vi "DataCollectWithTimeout.vi"(7 "Notifier Data":T2, 8 "error in (no error)":errorcluster, 9 "Timeout":dbl=5.0, 10 "Data Cluster":T1, 11 "Notifier in":refnum<notifier>) -> (0 "error out":errorcluster, 1 "Free Air Flow Data":dbl[][](array[numeric]), 2 "STOP Button Pressed":bool, 3 "Free Air Flow Measurement Complete":bool, 4 "Vacuum Data":dbl, 5 "Air Flow Data":dbl)   [LabVIEW 2026, in "Acquisition.lvlib"]
uses:
  Acquisition.lvlib
  controls/NotifierAndDataQueue.ctl
  controls/WaveformChartData.ctl
  Hardware Configuration.ctl
  Settings/Settings.lvlib
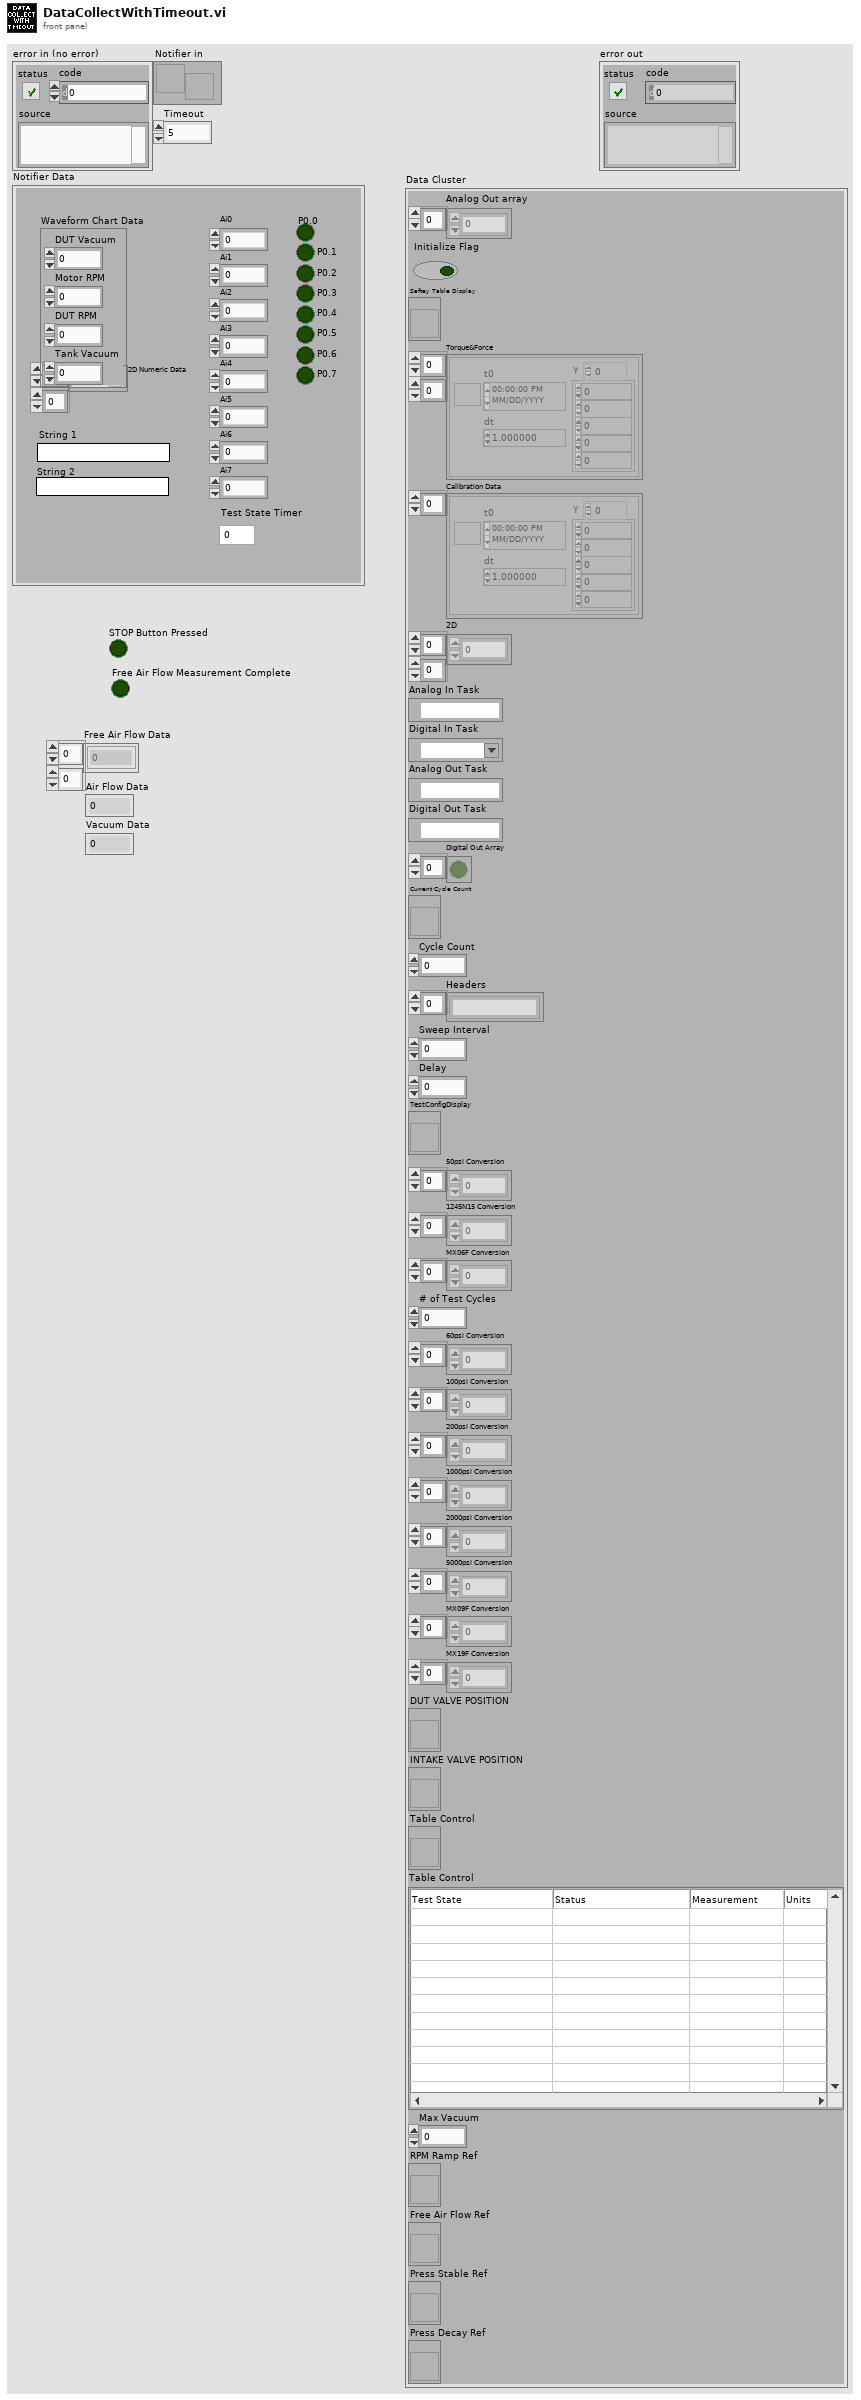
[diagram p1: front panel]
types:
  T1 = typedef "Acquisition.lvlib/Hardware Configuration.ctl" = cluster{"Analog Out array":dbl[], "Initialize Flag":bool, "Saftey Table Display":refnum<vi>, "Torque&Force":waveform(dbl)[][], "Calibration Data":waveform(dbl)[], "2D":dbl[][], "Analog In Task":refnum<k21>, "Digital In Task":refnum<k21>, "Analog Out Task":refnum<k21>, "Digital Out Task":refnum<k21>, "Digital Out Array":bool[], "Current Cycle Count":refnum<vi>, "Cycle Count":u64, "Headers":string[], "Sweep Interval":u64, "Delay":u64, "TestConfigDisplay":refnum<vi>, "50psi Conversion":dbl[], "1245N15 Conversion":dbl[], "MX06F Conversion":dbl[], "# of Test Cycles":u64, "60psi Conversion":dbl[], "100psi Conversion":dbl[], "200psi Conversion":dbl[], "1000psi Conversion":dbl[], "2000psi Conversion":dbl[], "5000psi Conversion":dbl[], "MX09F Conversion":dbl[], "MX19F Conversion":dbl[], "DUT VALVE POSITION":refnum<vi>, "INTAKE VALVE POSITION":refnum<vi>, "Table Control":refnum<vi>, "Table Control":string[][], "Max Vacuum":dbl, "RPM Ramp Ref":refnum<vi>, "Free Air Flow Ref":refnum<vi>, "Press Stable Ref":refnum<vi>, "Press Decay Ref":refnum<vi>}
  T2 = typedef "NotifierAndDataQueue.ctl" = cluster{"Ai0":dbl, "Ai1":dbl, "Ai2":dbl, "Ai3":dbl, "Ai4":dbl, "Ai5":dbl, "Ai6":dbl, "Ai7":dbl, "P0.0":bool, "P0.1":bool, "P0.2":bool, "P0.3":bool, "P0.4":bool, "P0.5":bool, "P0.6":bool, "P0.7":bool, "2D Numeric Data":dbl[][], "String 2":string, "String 1":string, "Waveform Chart Data":T3, "Test State Timer":dbl}
  T3 = typedef "Settings.lvlib/WaveformChartData.ctl" = cluster{"DUT Vacuum":dbl, "Motor RPM":dbl, "DUT RPM":dbl, "Tank Vacuum":dbl}
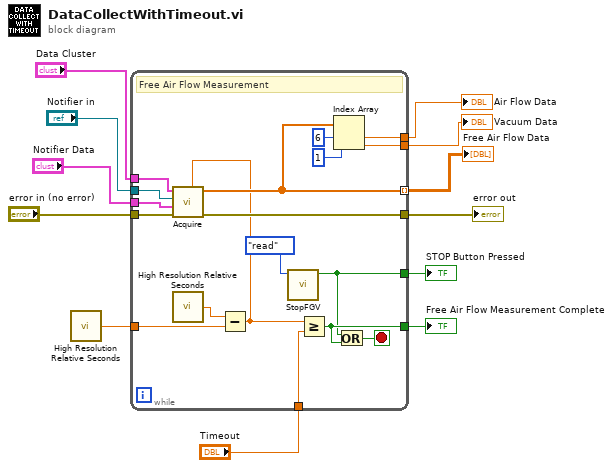
[diagram p0: block diagram]
diagram:
  n1 = call <vilib>:"High Resolution Relative Seconds.vi"() -> ("relative seconds"=w5:dbl)
  n2 = while {
    tunnel: "Notifier in" -> [w28]
    tunnel: "error in (no error)" -> [w30]
    tunnel: [w29] -> w9
    tunnel: "Notifier Data" -> [w25]
    tunnel: "Data Cluster" -> [w24]
    tunnel: [w21] -> w7
    tunnel: [w22] -> w6
    tunnel: w5 -> [w20]
    tunnel: [w18] -> w4 mode=indexing
    tunnel: "Timeout" -> [w19]
    tunnel: [w17] -> w2
    tunnel: [w14] -> w1
    stop <- w26 stop-if-true
    # "Free Air Flow Measurement"
    n3 = call <vilib>:"High Resolution Relative Seconds.vi"() -> ("relative seconds"=w23:dbl)
    n4 = Subtract(x=w23, y=w20) -> (x-y=w13:dbl)
    n5 = call "Acquire.vi"("Test State Timer"=w13, "error in (no error)"=w30, "Notifiier Data"=w25, "notifier out"=w28, "Hardware Resources in"=w24) -> ("error out"=w29:errorcluster, "Averaged Data Array"=w18:dbl[])  [unwired: 4 in, 1 out]
    n6 = call "StopFGV.vi"("Enum"=enum16{"init", "write", "read"}."read") -> ("STOP Out"=w21:bool)  [unwired: 9 in, 1 out]
    n7 = Greater Or Equal?(x=w13, y=w19) -> (x >= y?=w22:bool)
    n8 = Index Array(array=w18, index #1=6 ("index"), index #2=1 ("index")) -> (element #1=w17:dbl, element #2=w14:dbl)
    n9 = Or(x=w21, y=w22) -> (x .or. y?=w26:bool)
  }
  "error out" <- w9
  "STOP Button Pressed" <- w7
  "Free Air Flow Measurement Complete" <- w6
  "Free Air Flow Data" <- w4
  "Air Flow Data" <- w2
  "Vacuum Data" <- w1
